vi "Funct TIFF export-Core.vi"(8 "error in (no error)":errorcluster, 10 "ProgressBar":refnum<k24>, 11 "Info indicators only (F)":bool) -> ()   [LabVIEW 2013]
uses:
  System.Windows.Forms
  Globals/gl_funct TIFF export globals.vi
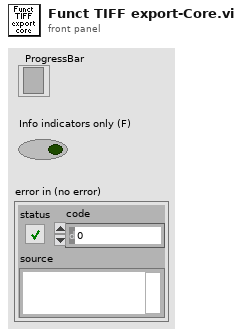
[diagram p1: front panel]
types:
  T1 = typedef "Funct TIFF exporter ctrl refs.ctl" = cluster{"This VI":refnum<vi>, "Current Experiment":refnum<vi>, "Imaging protocol":refnum<vi>, "Predominant ROI type":refnum<vi>, "Patches in Experiment":refnum<vi>, "Folder Path":refnum<vi>, "Export":refnum<vi>, "Trial number":refnum<vi>, "Output TIFF type":refnum<vi>}
  T2 = typedef "ROI ID Enum.ctl" = enum16{"Point", "MiniScan", "Comp. MiniScan", "Rectangle", "Comp. volume", "Arb. plane point"}
  T3 = typedef "Imaging Protocols enum.ctl" = enum16{"AOL Z-Stack", "Motor Z Stack", "Functional Acquisition", "Single Plane Acquisition", "Volume Acquisition", "Live Imaging", "Live Plane Imaging", "Live Volume Imaging"}
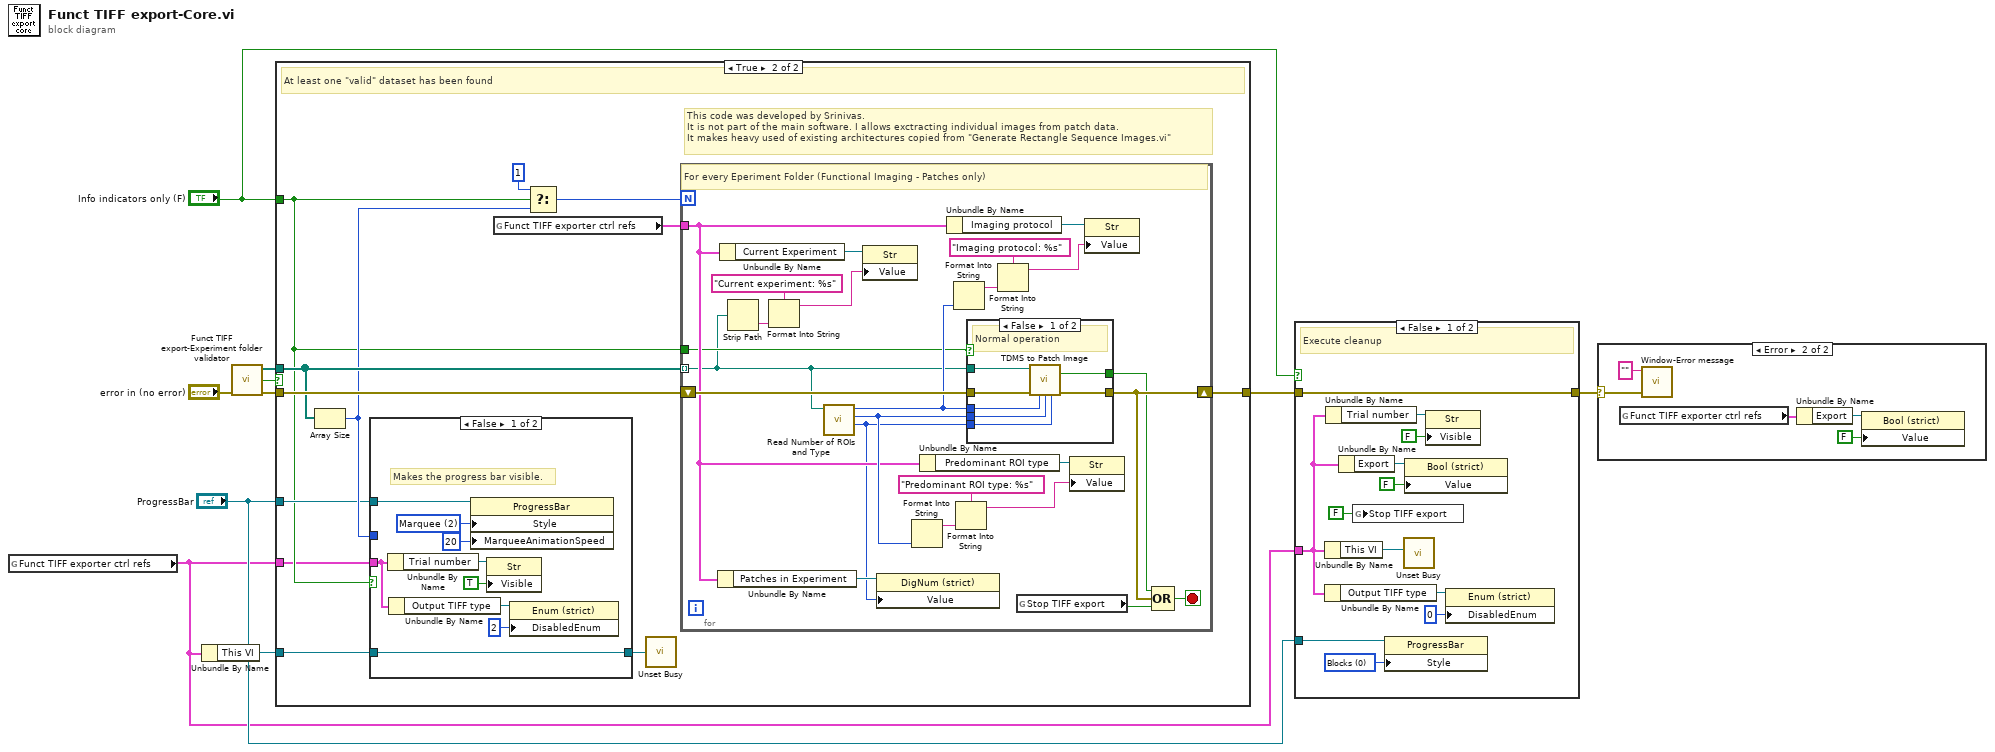
[diagram p0: block diagram]
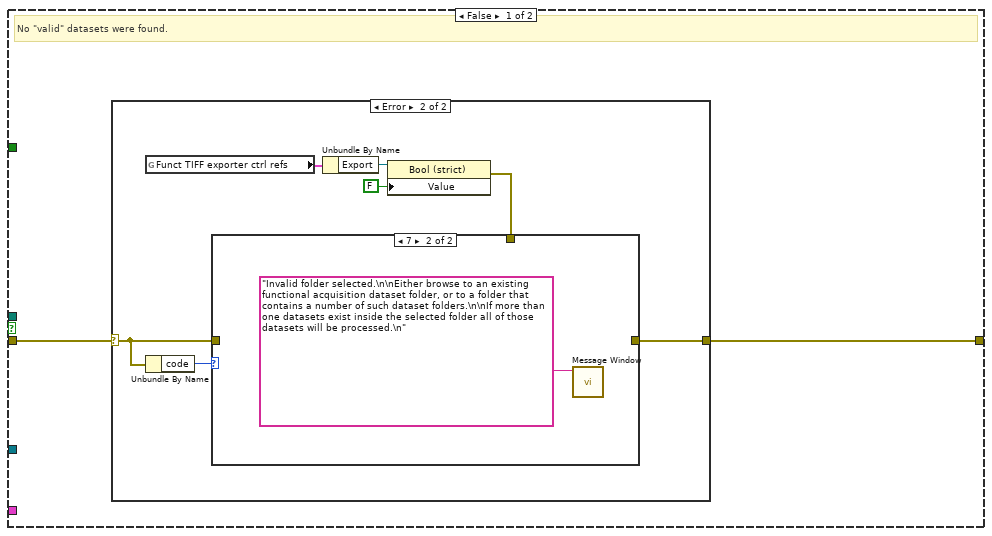
[diagram p4: hidden frame]
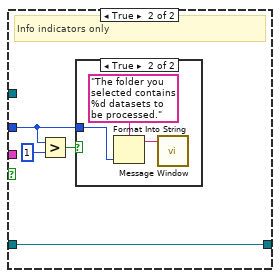
[diagram p7: hidden frame]
diagram:
  n1 = global read "gl_funct TIFF export globals.vi" "Funct TIFF exporter ctrl refs"() -> (w3:T1)
  n2 = Unbundle By Name(w3) -> ("This VI"=w6:refnum<vi>)
  n3 = call "Funct TIFF export-Experiment folder validator.vi"("error in (no error)"="error in (no error)") -> ("error out"=w10:errorcluster, "Valid experiment folders found"=w7:bool, "Filtered Array out"=w8:path[])  [unwired: 8 in]
  n4 = case shown="True" w7 {
    tunnel: w10 -> [w12 w34]
    tunnel: "Info indicators only (F)" -> [_ w24]
    tunnel: [w11 w31] -> w2
    tunnel: w8 -> [_ w29]
    tunnel: w6 -> [_ w27]
    tunnel: "ProgressBar" -> [_ w25]
    tunnel: w3 -> [_ w23]
    frame False {
      # "No \"valid\" datasets were found."
      n5 = case shown="Error" w12 {
        selector: w12 -> [w13 w19]
        tunnel: [w13 w18] -> w11
        frame No Error {
        }
        frame Error {
          n6 = global read "gl_funct TIFF export globals.vi" "Funct TIFF exporter ctrl refs"() -> (w17:T1)
          n7 = Unbundle By Name(w19) -> ("code"=w20:i32)
          n8 = Unbundle By Name(w17) -> ("Export"=w16:refnum<vi>)
          n9 = property class="Bool (strict)"(reference=w16, "Value"=FALSE) -> (error out=w14:errorcluster)  [unwired: 1 in, 1 out]
          n10 = case shown="7" w20 {
            tunnel: [w21 _] -> w18
            tunnel: w19 -> [w21 _]
            tunnel: w14 -> [_ _]
            frame 0, Default {
            }
            frame 7 {
              n11 = call "Message Window.vi"("Message string"="Invalid folder selected.\n\nEither browse to an existing functional acquisition dataset folder, or to a folder that contains a number of such dataset folders.\n\nIf more than one datasets exist inside the selected folder all of those datasets will be processed.\n") -> ()  [unwired: 10 in, 1 out]
            }
          }
        }
      }
    }
    frame True {
      # "This code was developed by Srinivas.\nIt is not part of the main software. I allows exctracting individual images from patch data.\nIt makes heavy used of existing architectures copied from \"Generate Rectangle Sequence Images.vi\""
      # "At least one \"valid\" dataset has been found"
      n12 = Array Size(array=w29) -> (size(s)=w28:i32)
      n13 = case shown="False" w24 {
        tunnel: w28 -> [_ w45]
        tunnel: [w43 w44] -> w26
        tunnel: w27 -> [w43 w44]
        tunnel: w25 -> [w42 _]
        tunnel: w23 -> [w36 _]
        frame False {
          w41 = 2 items=["Blocks", "Continuous", "Marquee"] ("Style")
          # "Makes the progress bar visible."
          n14 = Unbundle By Name(w36) -> ("Trial number"=w39:refnum<vi>)
          n15 = Unbundle By Name(w36) -> ("Output TIFF type"=w37:refnum<vi>)
          n16 = property class="ProgressBar"(reference=w42, "Style"=w41, "MarqueeAnimationSpeed"=20) -> ()  [unwired: 1 in, 2 out]
          n17 = property class="Str"(reference=w39, "Visible"=TRUE) -> ()  [unwired: 1 in, 2 out]
          n18 = property class="Enum (strict)"(reference=w37, "DisabledEnum"=2) -> ()  [unwired: 1 in, 2 out]
        }
        frame True {
          # "Info indicators only"
          n19 = Greater?(x=w45, y=1) -> (0:w46:bool)
          n20 = case shown="True" w46 {
            tunnel: w45 -> [_ w50]
            frame False {
            }
            frame True {
              n21 = Format Into String(format string="The folder you selected contains %d datasets to be processed.", w50) -> (resulting string=w48:string)  [unwired: 2 in, 1 out]
              n22 = call "Message Window.vi"("Message string"=w48) -> ()  [unwired: 10 in, 1 out]
            }
          }
        }
      }
      n23 = global read "gl_funct TIFF export globals.vi" "Funct TIFF exporter ctrl refs"() -> (w30:T1)
      n24 = Select(t=1, s=w24, f=w28) -> (s? t:f=w32:i32)
      n25 = call <vilib>:"Unset Busy.vi"("VI reference (current VI)"=w26) -> ()  [unwired: 10 in, 1 out]
      n26 = for {
        N: w32 -> [_]
        tunnel: w29 -> [w53] mode=indexing
        tunnel: w30 -> [w59]
        tunnel: w24 -> [w57]
        shift-right: [w54] -> w31
        shift-left: w34 -> [w74]
        stop <- w56 stop-if-true
        # "For every Eperiment Folder (Functional Imaging - Patches only)"
        n27 = Unbundle By Name(w59) -> ("Patches in Experiment"=w60:refnum<vi>)
        n28 = Unbundle By Name(w59) -> ("Current Experiment"=w66:refnum<vi>)
        n29 = Strip Path(path=w53) -> (name=w52:string)  [unwired: 1 out]
        n30 = Format Into String(format string="Current experiment: %s", w52) -> (resulting string=w65:string)  [unwired: 2 in, 1 out]
        n31 = call "Read Number of ROIs and Type.vi"("Experimental Folder"=w53) -> ("Patches in Experiment"=w58:i32, "Predominant ROI type"=w67:T2, "Imaging Protocol"=w72:T3)  [unwired: 8 in]
        n32 = property class="Str"(reference=w66, "Value"=w65) -> ()  [unwired: 1 in, 2 out]
        n33 = property class="DigNum (strict)"(reference=w60, "Value"=w58) -> ()  [unwired: 1 in, 2 out]
        n34 = Format Into String(w67) -> (resulting string=w69:string)  [unwired: 3 in, 1 out]
        n35 = Unbundle By Name(w59) -> ("Predominant ROI type"=w62:refnum<vi>)
        n36 = Unbundle By Name(w59) -> ("Imaging protocol"=w64:refnum<vi>)
        n37 = Format Into String(w72) -> (resulting string=w71:string)  [unwired: 3 in, 1 out]
        n38 = Format Into String(format string="Predominant ROI type: %s", w69) -> (resulting string=w61:string)  [unwired: 2 in, 1 out]
        n39 = case shown="False" w57 {
          tunnel: [w81 w82] -> w54
          tunnel: w74 -> [w80 w82]
          tunnel: w72 -> [w79 _]
          tunnel: w67 -> [w78 _]
          tunnel: w58 -> [w77 _]
          tunnel: w53 -> [w76 _]
          tunnel: [w75 _] -> w51
          frame False {
            # "Normal operation"
            n40 = call "TDMS to Patch Image.vi"("Experiment Path"=w76, "error in (no error)"=w80, "Imaging Protocol"=w79, "Predominant ROI type"=w78, "No of Patches in Experiment"=w77) -> ("Cancelled"=w75:bool, "error out"=w81:errorcluster)  [unwired: 7 in, 2 out]
          }
          frame True {
            # "Info indicators only"
          }
        }
        n41 = Format Into String(format string="Imaging protocol: %s", w71) -> (resulting string=w63:string)  [unwired: 2 in, 1 out]
        n42 = global read "gl_funct TIFF export globals.vi" "Stop TIFF export"() -> (w55:bool)
        n43 = property class="Str"(reference=w62, "Value"=w61) -> ()  [unwired: 1 in, 2 out]
        n44 = property class="Str"(reference=w64, "Value"=w63) -> ()  [unwired: 1 in, 2 out]
        n45 = Compound Arithmetic op=OR(w51, w54, w55) -> (w56:bool)
      }
    }
  }
  n46 = case shown="False" "Info indicators only (F)" {
    tunnel: "ProgressBar" -> [w92 _]
    tunnel: w3 -> [w83 _]
    tunnel: w2 -> [w86 w95]
    tunnel: [w86 w95] -> w1
    frame False {
      w93 = 0 items=["Blocks", "Continuous", "Marquee"] ("Style")
      # "Execute cleanup"
      n47 = Unbundle By Name(w83) -> ("This VI"=w91:refnum<vi>)
      n48 = Unbundle By Name(w83) -> ("Output TIFF type"=w85:refnum<vi>)
      n49 = Unbundle By Name(w83) -> ("Trial number"=w87:refnum<vi>)
      n50 = Unbundle By Name(w83) -> ("Export"=w90:refnum<vi>)
      n51 = global write "gl_funct TIFF export globals.vi" "Stop TIFF export"(FALSE ("Stop TIFF export")) -> ()
      n52 = property class="ProgressBar"(reference=w92, "Style"=w93) -> ()  [unwired: 1 in, 2 out]
      n53 = call <vilib>:"Unset Busy.vi"("VI reference (current VI)"=w91) -> ()  [unwired: 10 in, 1 out]
      n54 = property class="Bool (strict)"(reference=w90, "Value"=FALSE ("Export")) -> ()  [unwired: 1 in, 2 out]
      n55 = property class="Str"(reference=w87, "Visible"=FALSE) -> ()  [unwired: 1 in, 2 out]
      n56 = property class="Enum (strict)"(reference=w85, "DisabledEnum"=0) -> ()  [unwired: 1 in, 2 out]
    }
    frame True {
      # "Info indicators only"
    }
  }
  n57 = case shown="Error" w1 {
    selector: w1 -> [_ w100]
    frame No Error {
    }
    frame Error {
      n58 = global read "gl_funct TIFF export globals.vi" "Funct TIFF exporter ctrl refs"() -> (w96:T1)
      n59 = call "Window-Error message.vi"("error in (no error)"=w100, "Message"="") -> ()  [unwired: 9 in, 1 out]
      n60 = Unbundle By Name(w96) -> ("Export"=w97:refnum<vi>)
      n61 = property class="Bool (strict)"(reference=w97, "Value"=FALSE) -> ()  [unwired: 1 in, 2 out]
    }
  }
